vi "4_2GraphChart_BTS.vi"() -> ()   [LabVIEW 2014]
panel:
  out "XY Circle Graph":cluster{dbl[], dbl[]}(graph)
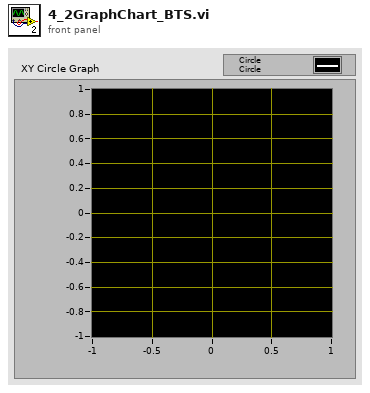
[diagram p1: front panel]
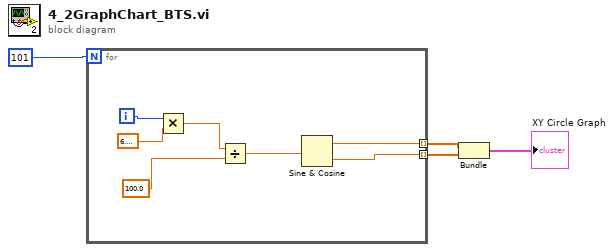
[diagram p0: block diagram]
diagram:
  n1 = for {
    N: 101 -> [_]
    tunnel: [w7] -> w3 mode=indexing
    tunnel: [w5] -> w2 mode=indexing
    i -> [w6]
    n2 = Multiply(x=w6, y=6.283185307179586) -> (x*y=w11:dbl)
    n3 = Divide(x=w11, y=100.0) -> (x/y=w8:dbl)
    n4 = Sine & Cosine(0:w8) -> (1:w7:dbl, 2:w5:dbl)
  }
  n5 = Bundle(w3, w2) -> (→"XY Circle Graph":cluster{dbl[], dbl[]})  [unwired: 1 in]
